vi "Manual_Turret_Control_untested.vi"() -> ()   [LabVIEW 2019]
uses:
  Control 4.ctl
panel:
  in  "Stop":dbl
  in  "Counter-Clockwise_Rotate":dbl
  in  "Clockwise_Rotate":dbl
  in  "Rotate_Counter-Clockwise":bool
  in  "Rotate_Clockwise":bool
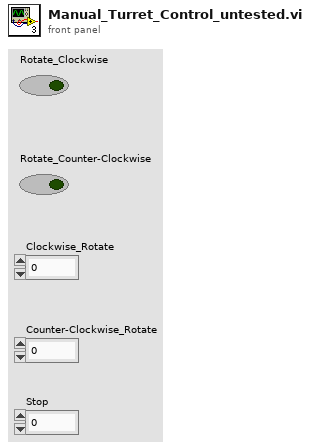
[diagram p1: front panel]
types:
  T1 = typedef "Control 4.ctl" = enum16{"Stop", "Rotate_Clockwise", "Rotate_Counter-Clockwise"}
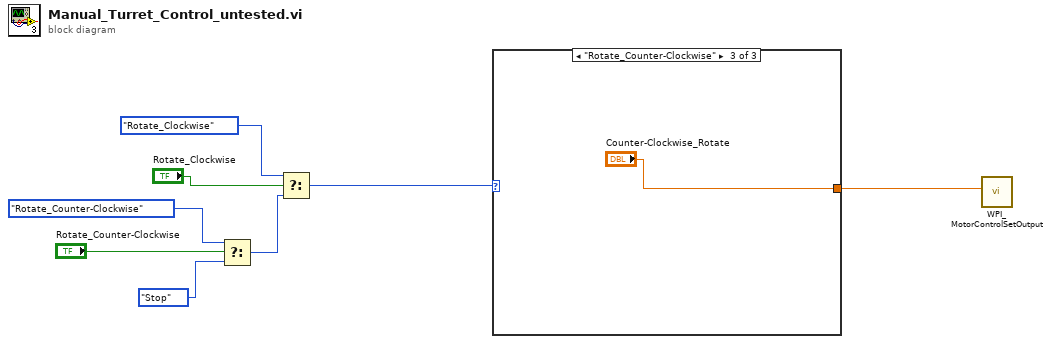
[diagram p0: block diagram]
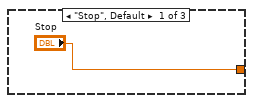
[diagram p2: hidden frame]
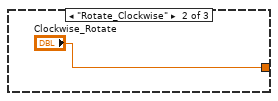
[diagram p3: hidden frame]
diagram:
  n1 = Select(t=Control_4."Rotate_Counter-Clockwise", s="Rotate_Counter-Clockwise", f=Control_4."Stop") -> (s? t:f=w6:T1)
  n2 = Select(t=Control_4."Rotate_Clockwise", s="Rotate_Clockwise", f=w6) -> (s? t:f=w2:T1)
  n3 = case shown="\"Rotate_Counter-Clockwise\"" w2 {
    tunnel: ["Stop" "Clockwise_Rotate" "Counter-Clockwise_Rotate"] -> w1
    frame "Stop", Default {
    }
    frame "Rotate_Clockwise" {
    }
    frame "Rotate_Counter-Clockwise" {
    }
  }
  n4 = call <vilib>:"WPI_MotorControlSetOutput.vi"("Output"=w1) -> ()  [unwired: 8 in, 3 out]
